vi "remove duplicate classes.vi"(8 "error in":errorcluster, 9 "class paths in":path[](array[path]), 10 "class names in":string[](array[string]), 11 "discovered classes":path[](array[path])) -> (0 "error out":errorcluster, 1 "class paths out":path[](array[path]), 2 "class names out":string[](array[string]))   [LabVIEW 2013, in "class discovery singleton.lvlib"]
uses:
  class discovery singleton.lvlib
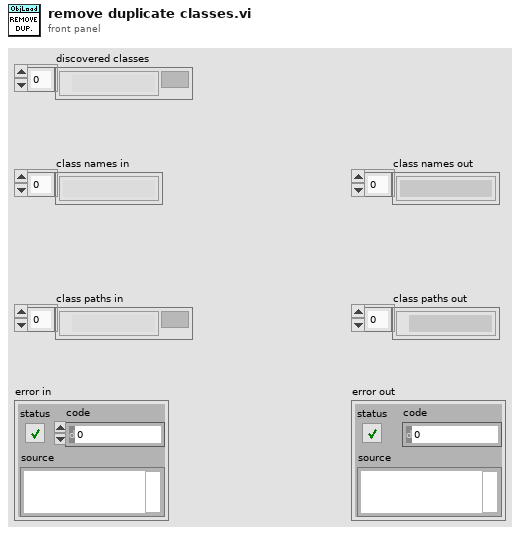
[diagram p1: front panel]
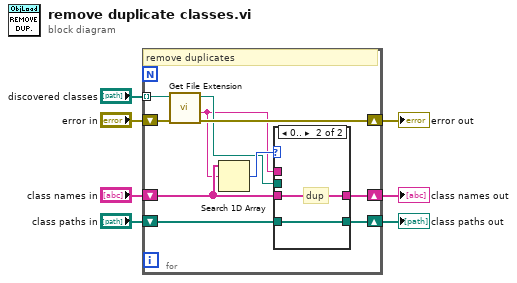
[diagram p0: block diagram]
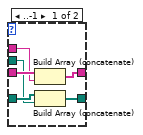
[diagram p2: hidden frame]
diagram:
  n1 = for {
    tunnel: "discovered classes" -> [w16] mode=indexing
    shift-right: [w15] -> w7
    shift-left: "error in" -> [w17]
    shift-right: [w11] -> w6
    shift-left: "class names in" -> [w13]
    shift-right: [w10] -> w5
    shift-left: "class paths in" -> [w12]
    # "remove duplicates"
    n2 = call <vilib>:"Get File Extension.vi"("error in (no error)"=w17, "file"=w16) -> ("error out"=w15:errorcluster, "filename without extension"=w8:string, "dup file"=w9:path)  [unwired: 6 in, 1 out]
    n3 = Search 1D Array(1D array=w13, element=w8) -> (index of element=w14:i32)  [unwired: 1 in]
    n4 = case shown="0.." w14 {
      tunnel: w13 -> [w21 w25]
      tunnel: w12 -> [w23 w24]
      tunnel: [w20 w25] -> w11
      tunnel: [w22 w24] -> w10
      tunnel: w9 -> [w19 _]
      tunnel: w8 -> [w18 _]
      frame ..-1 {
        n5 = Build Array (concatenate)(w21, w18) -> (w20:string[])
        n6 = Build Array (concatenate)(w23, w19) -> (w22:path[])
      }
      frame 0.. {
        # "dup"
      }
    }
  }
  "error out" <- w7
  "class names out" <- w6
  "class paths out" <- w5
